vi "Revision Query.vi"(8 "error in (no error)":errorcluster) -> (0 "error out":errorcluster, 1 "Instrument Version and Software Revision":string, 2 "Instrument Driver Revision":string)   [LabVIEW 2017, in "HighFinesse WS5.lvlib"]
doc: "Queries the current instrument name, serial number, and software revision, along with the instrument driver revision.\n\nRefer to the Readme file for detailed driver information including modification history."
uses:
  HighFinesse WS5.lvlib
  wlmData.dll
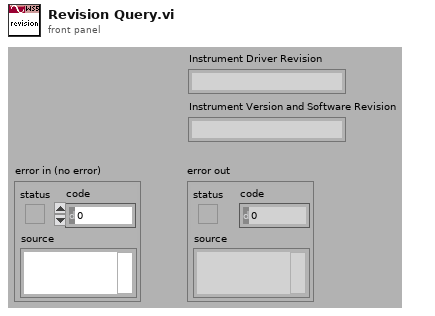
[diagram p1: front panel]
types:
  T1 = cluster{"Major":u16, "Minor":u16, "Fix":u16, "Build":u16}
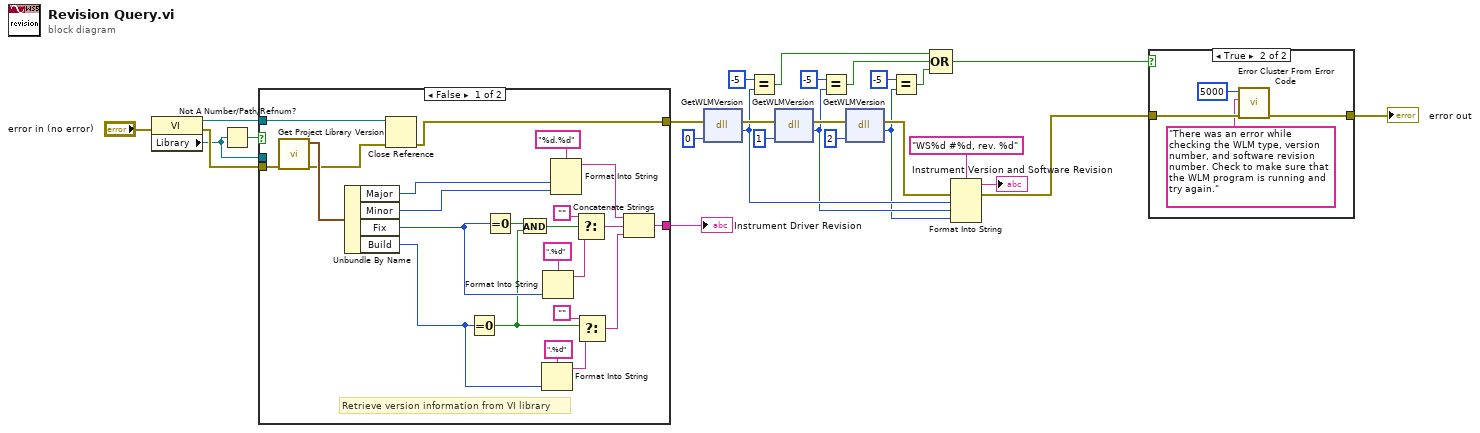
[diagram p0: block diagram]
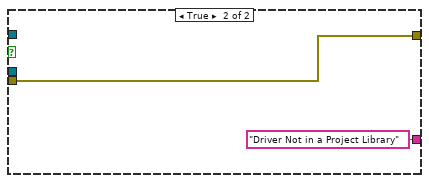
[diagram p2: hidden frame]
diagram:
  n1 = property class="VI"(error in="error in (no error)") -> (reference out=w4:refnum<vi>, error out=w3:errorcluster, "Library"=w2:refnum<vi>)  [unwired: 1 in]
  n2 = Not A Number/Path/Refnum?(number/path/refnum=w2) -> (NaN/Path/Refnum?=w1:bool)
  n3 = case shown="False" w1 {
    tunnel: w4 -> [w50 _]
    tunnel: w3 -> [w30 w52]
    tunnel: [w32 w52] -> w24
    tunnel: [w31 "Driver Not in a Project Library"] -> w27
    tunnel: w2 -> [_ _]
    frame False {
      # "Retrieve version information from VI library"
      n4 = call <vilib>:"Get Project Library Version.vi"("error in (no error)"=w30) -> ("error out"=w28:errorcluster, "Project Library Version"=w29:T1)  [unwired: 9 out]
      n5 = Unbundle By Name(w29) -> ("Major"=w39:u16, "Minor"=w38:u16, "Fix"=w36:u16, "Build"=w37:u16)
      n6 = Close Reference(reference=w50, error in (no error)=w28) -> (error out=w32:errorcluster)
      n7 = Equal To 0?(x=w37) -> (x = 0?=w34:bool)
      n8 = Equal To 0?(x=w36) -> (x = 0?=w35:bool)
      n9 = And(x=w35, y=w34) -> (x .and. y?=w33:bool)
      n10 = Format Into String(format string=".%d", w37) -> (resulting string=w43:string)  [unwired: 2 in, 1 out]
      n11 = Format Into String(format string=".%d", w36) -> (resulting string=w47:string)  [unwired: 2 in, 1 out]
      n12 = Format Into String(format string="%d.%d", w39, w38) -> (resulting string=w45:string)  [unwired: 2 in, 1 out]
      n13 = Select(t="", s=w33, f=w47) -> (s? t:f=w44:string)
      n14 = Select(t="", s=w34, f=w43) -> (s? t:f=w40:string)
      n15 = Concatenate Strings(w45, w44, w40) -> (w31:string)
    }
    frame True {
    }
  }
  "Instrument Driver Revision" <- w27
  n16 = dll-call lib="C:/LabVIEW-programs/Instruments/Wavelength meter/HighFinesse WS5/wlmData.dll" fn="GetWLMVersion"(error in=w24, "Ver"=0) -> (error out=w20:errorcluster, "return type"=w7:i32)  [unwired: 3 in, 1 out]
  n17 = Equal?(x=-5, y=w7) -> (x = y?=w12:bool)
  n18 = dll-call lib="C:/LabVIEW-programs/Instruments/Wavelength meter/HighFinesse WS5/wlmData.dll" fn="GetWLMVersion"(error in=w20, "Ver"=1) -> (error out=w18:errorcluster, "return type"=w6:i32)  [unwired: 3 in, 1 out]
  n19 = Equal?(x=-5, y=w6) -> (x = y?=w11:bool)
  n20 = dll-call lib="C:/LabVIEW-programs/Instruments/Wavelength meter/HighFinesse WS5/wlmData.dll" fn="GetWLMVersion"(error in=w18, "Ver"=2) -> (error out=w13:errorcluster, "return type"=w5:i32)  [unwired: 3 in, 1 out]
  n21 = Equal?(x=-5, y=w5) -> (x = y?=w10:bool)
  n22 = Compound Arithmetic op=OR(w12, w11, w10) -> (w8:bool)
  n23 = Format Into String(format string="WS%d #%d, rev. %d", error in=w13, w7, w6, w5) -> (resulting string=→"Instrument Version and Software Revision":string, error out=w9:errorcluster)  [unwired: 1 in]
  n24 = case shown="True" w8 {
    tunnel: w9 -> [w53 w57]
    tunnel: [w53 w55] -> w23
    frame False {
    }
    frame True {
      n25 = call <vilib>:"Error Cluster From Error Code.vi"("error in (no error)"=w57, "error message (\"\")"="There was an error while checking the WLM type, version number, and software revision number. Check to make sure that the WLM program is running and try again." ("error source (\" \")"), "error code (0)"=5000 ("error code (no error:0)")) -> ("error out"=w55:errorcluster)  [unwired: 2 in, 4 out]
    }
  }
  "error out" <- w23
